vi "ReCalc_V0.11.vi"() -> ()   [LabVIEW 2014]
uses:
  <vilib>/Utility/miscctls.llb/LVPointTypeDef.ctl
  <vilib>/Utility/NIReport.llb/Append Report Text (str wrap).vi
  <vilib>/Utility/xml.llb/Write to XML File(string).vi
  <vilib>/Utility/xml.llb/Read From XML File(string).vi
  <vilib>/Analysis/3filter.llb/IIR Filter (DBL).vi
  <vilib>/Utility/NIReport.llb/NI_report.lvclass
  <vilib>/Analysis/NI_AALPro.lvlib
  <vilib>/Analysis/NI_AALBase.lvlib
panel:
  out "Übersetzung ermitteln aus":T1(ring)
  in  "Datenspeicher":T2
  in  "Speichern":bool
  out "Reifenumfang [m]":dbl=1.222
  out "Getriebe [1:]":dbl=5.343
  out "Zündung [Imp/U]":u8=1
  out "Rolle [Inkr/U]":u16=200
  out "Luftdruck [mbar]":dbl=1013.0
  out "Luftfeuchtigkeit [%]":dbl=50.0
  out "Lufttemperatur [°C]":dbl=20.0
  in  "Berechnen":bool
  in  "Stopp":bool
  in  "Rollenträgheit [kgm²]":dbl=0.402
  in  "Polynom":u8=15
  in  "Gl. Mittelwert":u8=35
  in  "Differenzenquotient":u8=12
  in  "n vom Gas [1/min]":dbl=5000.0
  out "Rollenumfang [m]":dbl=0.613 format="%.3f"
  out "Datum, Zeit":string
  out "Untersetzung aus:":dbl=2.68 format="%.2f"
  in  "Drucken":bool
  out "Pmax":string
  out "Ergebnis":string
  out "Fahrzeugdaten":string
  out "XY-Graph":cluster{dbl[], dbl[]}[](graph)
  in  "Öffnen":bool
  out "korr":dbl
  out "[s]":dbl=5.0
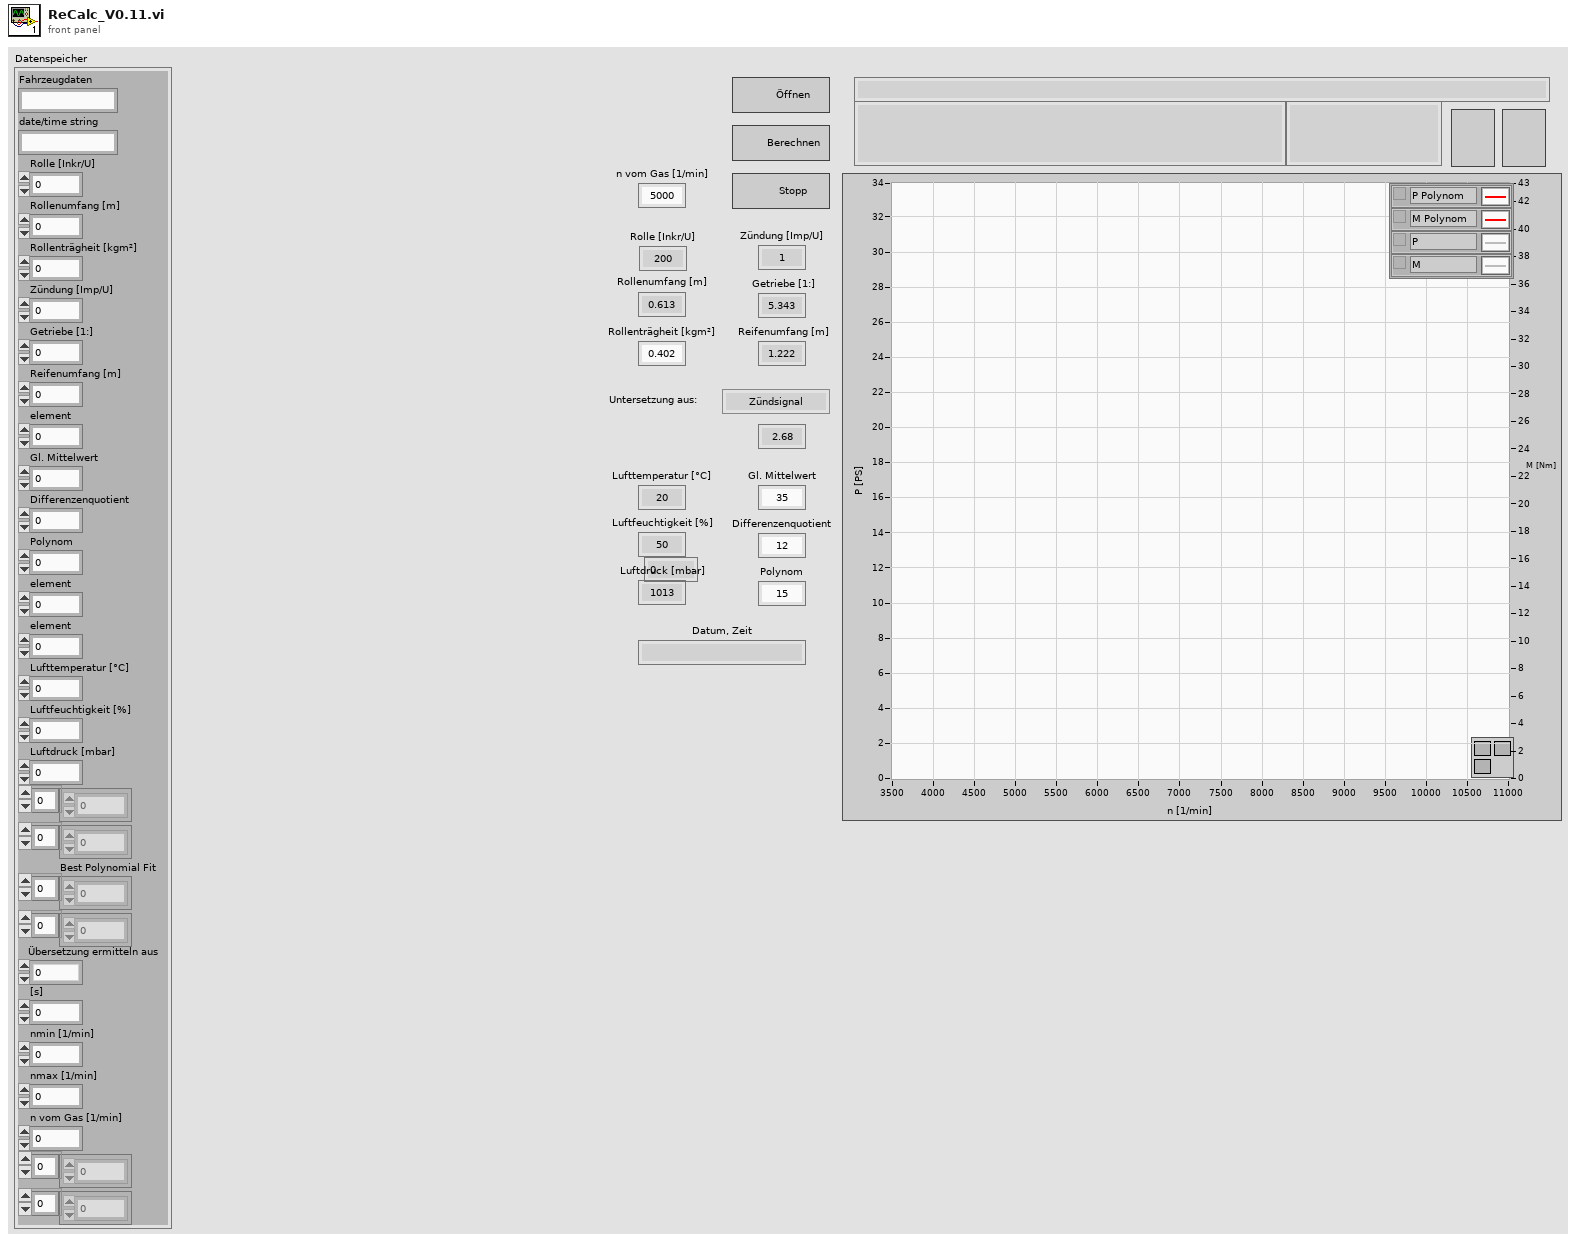
[diagram p1: front panel]
types:
  T1 = enum8{"Zündsignal", "Getriebe & Reifen", "nKuWe / nRolle :"}
  T2 = cluster{"Fahrzeugdaten":string, "date/time string":string, "Rolle [Inkr/U]":u16, "Rollenumfang [m]":dbl, "Rollenträgheit [kgm²]":dbl, "Zündung [Imp/U]":u8, "Getriebe [1:]":dbl, "Reifenumfang [m] ":dbl, "element":dbl, "Gl. Mittelwert":u8, "Differenzenquotient":u8, "Polynom":u8, "element":dbl, "element":dbl, "Lufttemperatur [°C]":dbl, "Luftfeuchtigkeit [%]":dbl, "Luftdruck [mbar]":dbl, dbl[], dbl[], "Best Polynomial Fit":dbl[], dbl[], "Übersetzung ermitteln aus":u8, "[s]":dbl, "nmin [1/min]":dbl, "nmax [1/min]":dbl, "n vom Gas [1/min]":dbl, dbl[], i32[]}
  T3 = typedef "LVPointTypeDef.ctl" = cluster{"Horizontal":i16, "Vertical":i16}
  T4 = enum16{"Kleinste Quadrate", "Kleinestes absolutes Reiduum", "Biquadrat"}
  T5 = cluster{"Fahrzeugdaten":string, "Value":string, "Value":u16, "Value":dbl, "Value":dbl, "Value":u8, "Value":dbl, "Value":dbl, "Value":dbl, "Value":u8, "Value":u8, "Value":u8, "element":dbl, "element":dbl, "Value":dbl, "Value":dbl, "Value":dbl, dbl[], dbl[], "Best Polynomial Fit":dbl[], dbl[], u8, "Value":dbl, dbl, dbl, "Value":dbl, dbl[], i32[]}
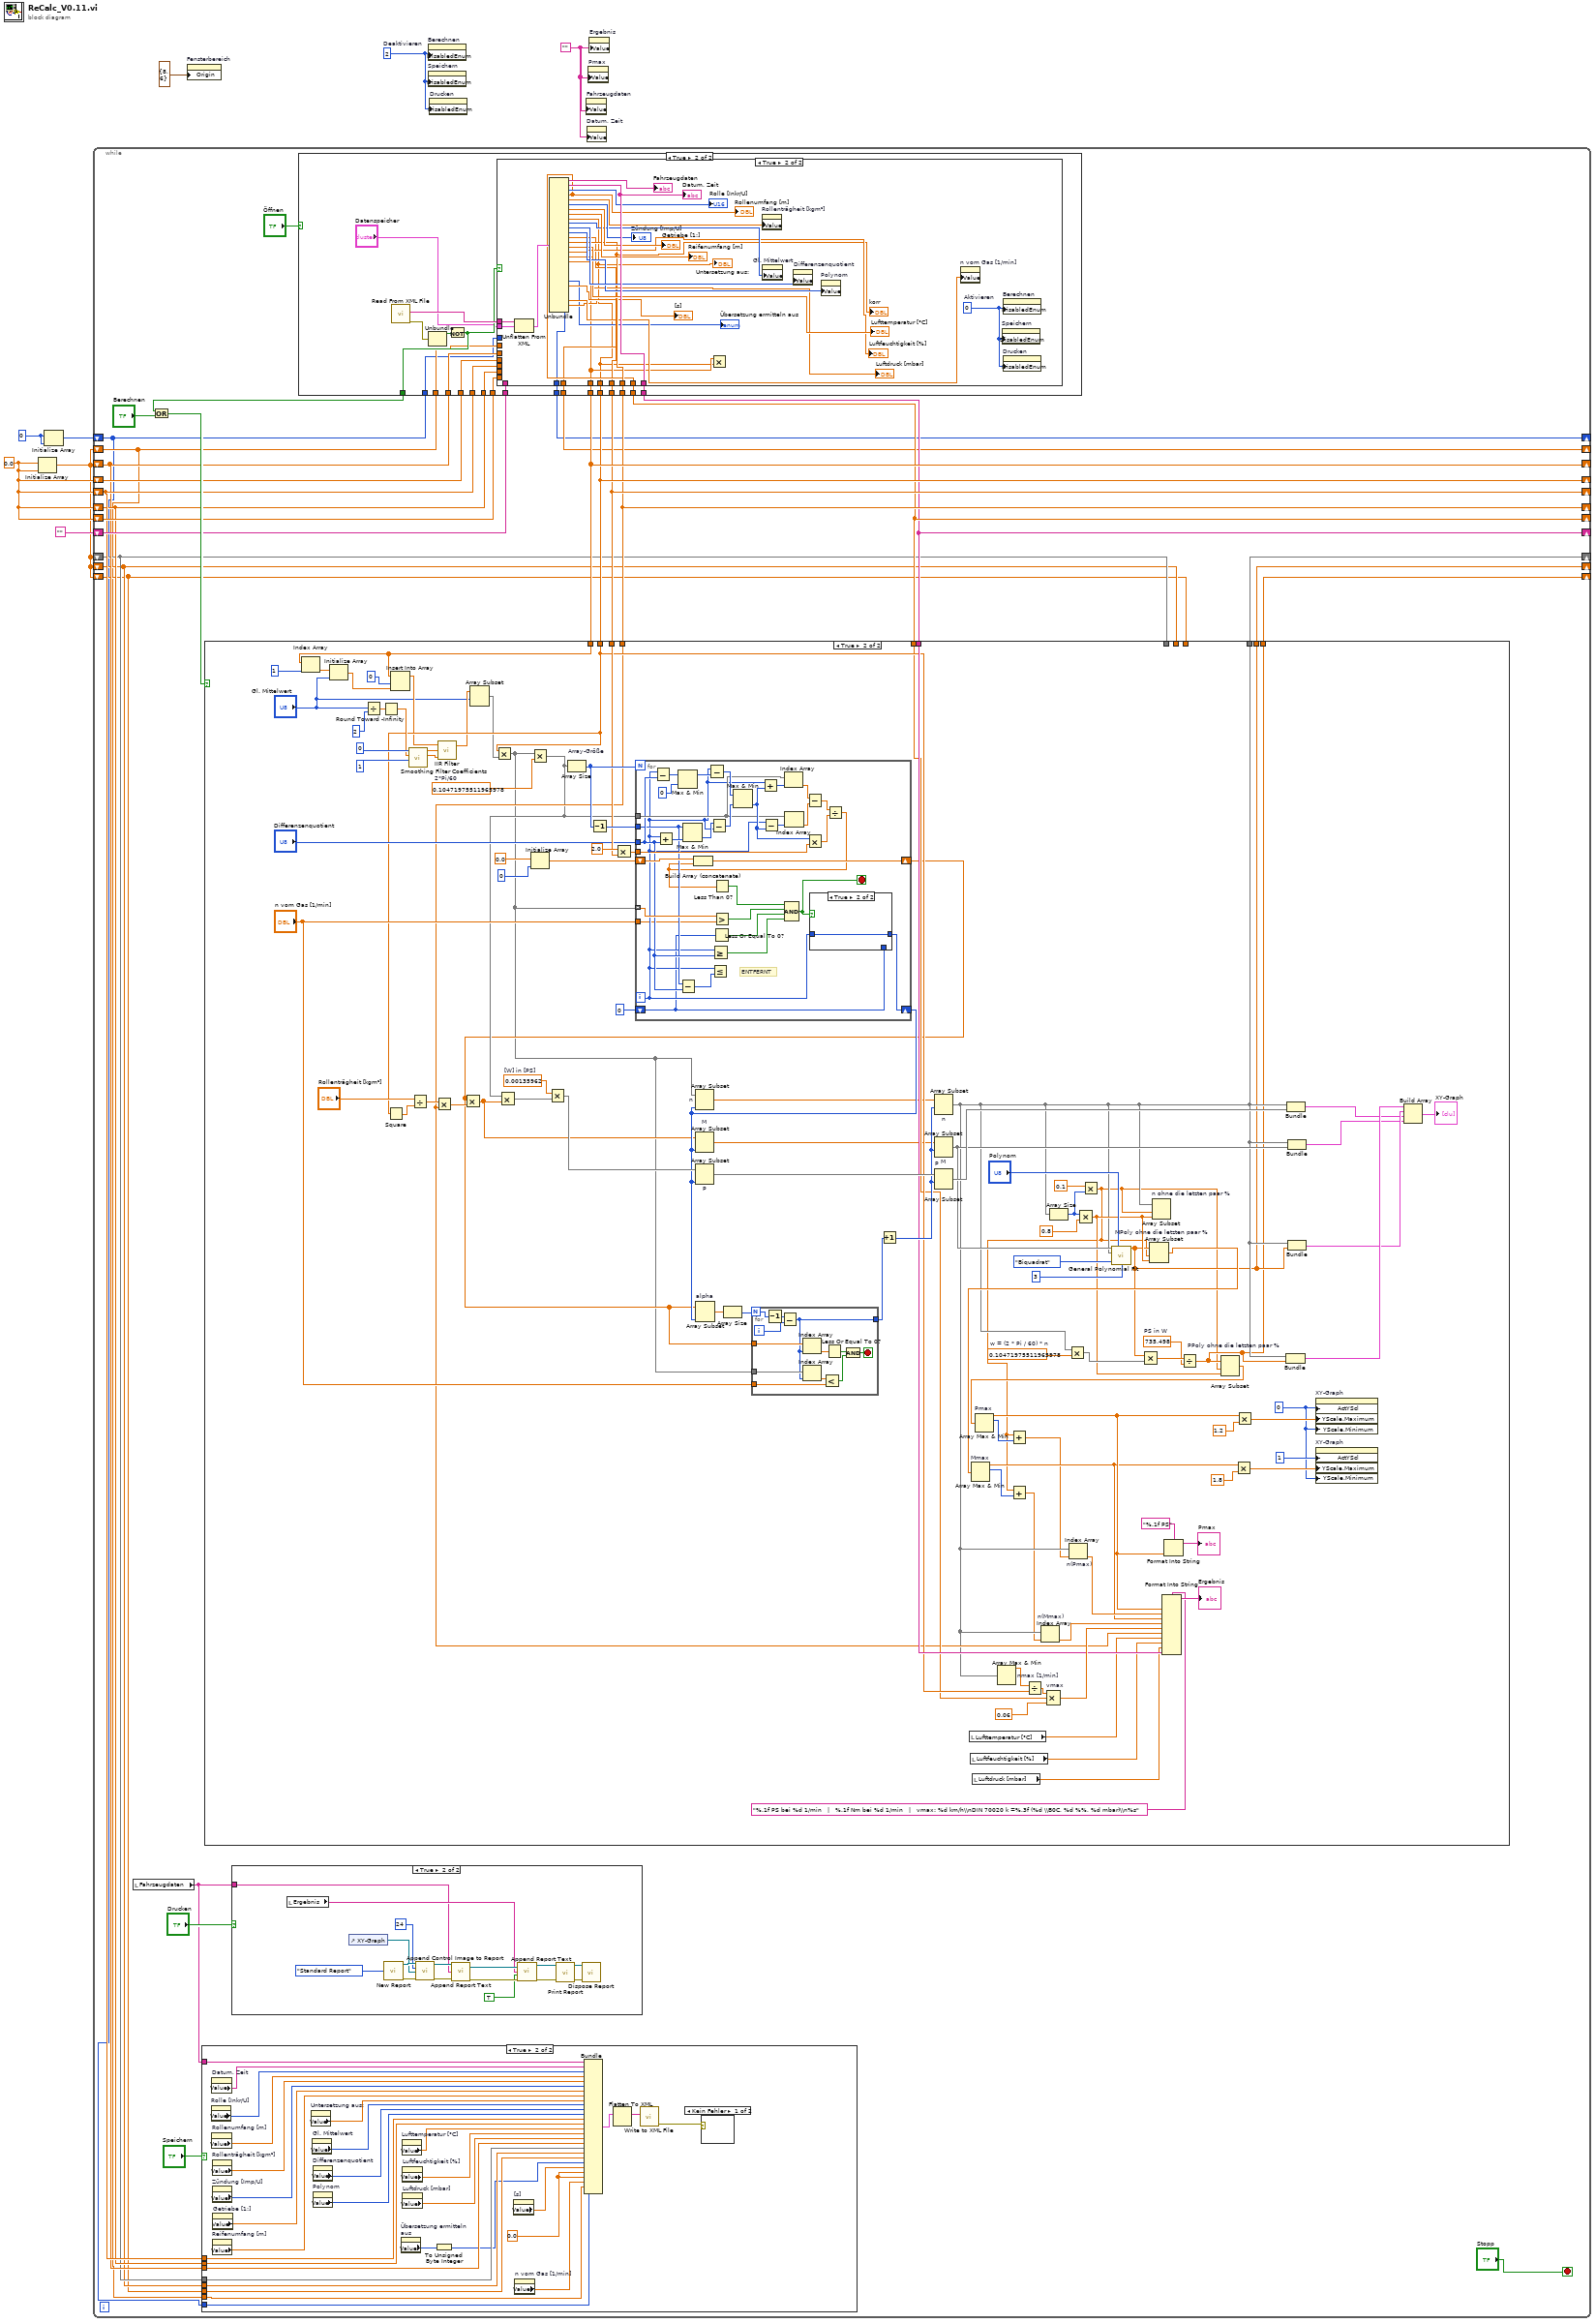
[diagram p0: block diagram]
diagram:
  w1 = 0
  w7 = 0.0
  w4 = 2  # Deaktivieren
  w8 = ""
  n1 = Initialize Array(w7, w7) -> (w3:dbl[])
  n2 = Initialize Array(w1, w1) -> (w2:i32[])
  n3 = while {
    shift-right: [w30] -> _
    shift-left: w3 -> [w19]
    shift-right: [w29] -> _
    shift-left: w7 -> [w33]
    shift-right: [w28] -> _
    shift-left: w7 -> [w21]
    shift-right: [w27] -> _
    shift-left: w7 -> [w20]
    shift-right: [w26] -> _
    shift-left: w7 -> [w32]
    shift-right: [w25] -> _
    shift-left: "" -> [w31]
    shift-right: [w18] -> _
    shift-left: w3 -> [w15]
    shift-right: [w17] -> _
    shift-left: w3 -> [w14]
    shift-right: [w16] -> _
    shift-left: w3 -> [w13]
    shift-right: [w12] -> _
    shift-left: w3 -> [w11]
    shift-right: [w10] -> _
    shift-left: w2 -> [w9]
    stop <- "Stopp" stop-if-true
    n4 = local read "Fahrzeugdaten"() -> (w22:string)
    n5 = case shown="True" "Speichern" {
      tunnel: w22 -> [_ w67]
      tunnel: w21 -> [_ w55]
      tunnel: w20 -> [_ w54]
      tunnel: w19 -> [_ w50]
      tunnel: w15 -> [_ w49]
      tunnel: w14 -> [_ w48]
      tunnel: w13 -> [_ w47]
      tunnel: w11 -> [_ w43]
      tunnel: w9 -> [_ w42]
      frame False {
      }
      frame True {
        w41 = 0.0
        n6 = property on="Rolle [Inkr/U]" class="DigWert (strikt)"() -> ("Value"=w65:u16)  [unwired: 2 in, 2 out]
        n7 = property on="Datum, Zeit" class="Str"() -> ("Value"=w66:string)  [unwired: 2 in, 2 out]
        n8 = property on="Rollenumfang [m]" class="DigWert (strikt)"() -> ("Value"=w64:dbl)  [unwired: 2 in, 2 out]
        n9 = property on="Rollenträgheit [kgm²]" class="DigWert (strikt)"() -> ("Value"=w63:dbl)  [unwired: 2 in, 2 out]
        n10 = property on="Zündung [Imp/U]" class="DigWert (strikt)"() -> ("Value"=w62:u8)  [unwired: 2 in, 2 out]
        n11 = property on="Reifenumfang [m]" class="DigWert (strikt)"() -> ("Value"=w60:dbl)  [unwired: 2 in, 2 out]
        n12 = property on="Getriebe [1:]" class="DigWert (strikt)"() -> ("Value"=w61:dbl)  [unwired: 2 in, 2 out]
        n13 = property on="Untersetzung aus:" class="DigWert (strikt)"() -> ("Value"=w59:dbl)  [unwired: 2 in, 2 out]
        n14 = property on="Gl. Mittelwert" class="DigWert (strikt)"() -> ("Value"=w58:u8)  [unwired: 2 in, 2 out]
        n15 = property on="Differenzenquotient" class="DigWert (strikt)"() -> ("Value"=w57:u8)  [unwired: 2 in, 2 out]
        n16 = property on="Polynom" class="DigWert (strikt)"() -> ("Value"=w56:u8)  [unwired: 2 in, 2 out]
        n17 = property on="Übersetzung ermitteln aus" class="Enum (strikt)"() -> ("Value"=w40:T1)  [unwired: 2 in, 2 out]
        n18 = property on="Lufttemperatur [°C]" class="DigWert (strikt)"() -> ("Value"=w53:dbl)  [unwired: 2 in, 2 out]
        n19 = property on="Luftfeuchtigkeit [%]" class="DigWert (strikt)"() -> ("Value"=w52:dbl)  [unwired: 2 in, 2 out]
        n20 = property on="Luftdruck [mbar]" class="DigWert (strikt)"() -> ("Value"=w51:dbl)  [unwired: 2 in, 2 out]
        n21 = To Unsigned Byte Integer(number=w40) -> (unsigned 8bit integer=w39:u8)
        n22 = property on="[s]" class="DigWert (strikt)"() -> ("Value"=w46:dbl)  [unwired: 2 in, 2 out]
        n23 = property on="n vom Gas [1/min]" class="DigWert (strikt)"() -> ("Value"=w45:dbl)  [unwired: 2 in, 2 out]
        n24 = Bundle("Fahrzeugdaten"=w67, "Value"=w66, "Value"=w65, "Value"=w64, "Value"=w63, "Value"=w62, "Value"=w61, "Value"=w60, "Value"=w59, "Value"=w58, "Value"=w57, "Value"=w56, "element"=w55, "element"=w54, "Value"=w53, "Value"=w52, "Value"=w51, w50, w49, "Best Polynomial Fit"=w48, w47, w39, "Value"=w46, w41, w41, "Value"=w45, w43, w42) -> (w68:T5)  [unwired: 1 in]
        n25 = Flatten To XML(anything=w68) -> (xml string=w69:string)
        n26 = call-poly <vilib>:"Write to XML File.vi"("XML Input"=w69) -> ("error out"=w44:errorcluster)  [unwired: 8 in, 2 out]
        n27 = case shown="Kein Fehler" w44 {
          frame No Error {
          }
          frame Error {
          }
        }
      }
    }
    n28 = case shown="True" "Drucken" {
      tunnel: w22 -> [_ w72]
      frame False {
      }
      frame True {
        n29 = local read "Ergebnis"() -> (w73:string)
        n30 = control-ref of="XY-Graph"() -> (w76:refnum<vi>)
        n31 = call <vilib>:"New Report.vi"("report type"=enum16{"Standard Report", "HTML"}."Standard Report") -> ("report out"=w85:refnum<class "NI_report.lvclass">, "error out"=w84:errorcluster)  [unwired: 13 in]
        n32 = call-dynamic "Append Control Image to Report.vi"("report in"=w85, "image depth"=24, "ctrl reference"=w76, "error in (no error)"=w84) -> ("report out"=w80:refnum<class "NI_report.lvclass">, "error out"=w81:errorcluster)  [unwired: 8 in, 2 out]
        n33 = call-poly <vilib>:"Append Report Text.vi"("report in"=w80, "text"=w72, "error in (no error)"=w81) -> ("report out"=w79:refnum<class "NI_report.lvclass">, "error out"=w78:errorcluster)  [unwired: 9 in, 2 out]
        n34 = call-poly <vilib>:"Append Report Text.vi"("report in"=w79, "text"=w73, "append on new line? (F)"=TRUE, "error in (no error)"=w78) -> ("report out"=w71:refnum<class "NI_report.lvclass">, "error out"=w70:errorcluster)  [unwired: 8 in, 2 out]
        n35 = call-dynamic "Print Report.vi"("report in"=w71, "error in (no error)"=w70) -> ("report out"=w82:refnum<class "NI_report.lvclass">, "error out"=w83:errorcluster)  [unwired: 12 in]
        n36 = call-dynamic "Dispose Report.vi"("report in"=w82, "error in (no error)"=w83) -> ()  [unwired: 13 in, 1 out]
      }
    }
    n37 = case shown="True" "Öffnen" {
      selector: "Öffnen" -> [w243 _]
      tunnel: [w242 w260] -> w30
      tunnel: [w241 w259] -> w29
      tunnel: [w240 w256] -> w28
      tunnel: [w239 w258] -> w27
      tunnel: [w243 w255] -> w37
      tunnel: [w237 w261] -> w25
      tunnel: [w238 w257] -> w26
      tunnel: w19 -> [w242 w254]
      tunnel: w33 -> [w241 w253]
      tunnel: w21 -> [w240 w252]
      tunnel: w20 -> [w239 w250]
      tunnel: w32 -> [w238 w251]
      tunnel: w31 -> [w237 w249]
      tunnel: w11 -> [w236 w248]
      tunnel: [w236 w247] -> w12
      tunnel: [w235 w246] -> w10
      tunnel: w9 -> [w235 w245]
      frame False {
      }
      frame True {
        n38 = call-poly <vilib>:"Read From XML File.vi"() -> ("error out"=w263:errorcluster, "XML Elements"=w264:string)  [unwired: 9 in, 1 out]
        n39 = Unbundle(w263) -> ("status"=w262:bool)  [unwired: 2 out]
        n40 = Not(x=w262) -> (.not. x?=w255:bool)
        n41 = case shown="True" w255 {
          tunnel: w264 -> [_ w299]
          tunnel: "Datenspeicher" -> [_ w298]
          tunnel: [w267 w295] -> w261
          tunnel: [w272 w274] -> w260
          tunnel: [w271 w273] -> w259
          tunnel: [w268 w283] -> w258
          tunnel: [w269 w282] -> w257
          tunnel: [w270 w281] -> w256
          tunnel: w254 -> [w272 _]
          tunnel: w253 -> [w271 _]
          tunnel: w252 -> [w270 _]
          tunnel: w251 -> [w269 _]
          tunnel: w250 -> [w268 _]
          tunnel: w249 -> [w267 _]
          tunnel: w248 -> [w266 _]
          tunnel: [w266 w277] -> w247
          tunnel: [w265 w276] -> w246
          tunnel: w245 -> [w265 _]
          frame False {
          }
          frame True {
            w278 = 0  # Aktivieren
            n42 = Unflatten From XML(xml string=w299, type=w298) -> (value=w297:T2)  [unwired: 1 in, 1 out]
            n43 = Unbundle(w297) -> ("Fahrzeugdaten"=→"Fahrzeugdaten":string, "date/time string"=w295:string, "Rolle [Inkr/U]"=→"Rolle [Inkr/U]":u16, "Rollenumfang [m]"=w282:dbl, "Rollenträgheit [kgm²]"=w292:dbl, "Zündung [Imp/U]"=→"Zündung [Imp/U]":u8, "Getriebe [1:]"=→"Getriebe [1:]":dbl, "Reifenumfang [m]"=→"Reifenumfang [m]":dbl, "element"=w273:dbl, "Gl. Mittelwert"=w289:u8, "Differenzenquotient"=w288:u8, "Polynom"=w287:u8, "element"=w281:dbl, "element"=w283:dbl, "Lufttemperatur [°C]"=→"Lufttemperatur [°C]":dbl, "Luftfeuchtigkeit [%]"=→"Luftfeuchtigkeit [%]":dbl, "Luftdruck [mbar]"=→"Luftdruck [mbar]":dbl, w274:dbl[], "Übersetzung ermitteln aus"=→"Übersetzung ermitteln aus":u8, "[s]"=→"[s]":dbl, "n vom Gas [1/min]"=w279:dbl, w277:dbl[], w276:i32[])  [unwired: 5 out]
            "Datum, Zeit" <- w295
            "Untersetzung aus:" <- w273
            "Rollenumfang [m]" <- w282
            "korr" <- w283
            n44 = Multiply(x=w274, y=w273) -> ()  [unwired: 1 out]
            n45 = property on="Rollenträgheit [kgm²]" class="DigWert (strikt)"("Value"=w292) -> ()  [unwired: 2 in, 2 out]
            n46 = property on="Gl. Mittelwert" class="DigWert (strikt)"("Value"=w289) -> ()  [unwired: 2 in, 2 out]
            n47 = property on="Differenzenquotient" class="DigWert (strikt)"("Value"=w288) -> ()  [unwired: 2 in, 2 out]
            n48 = property on="Polynom" class="DigWert (strikt)"("Value"=w287) -> ()  [unwired: 2 in, 2 out]
            n49 = property on="n vom Gas [1/min]" class="DigWert (strikt)"("Value"=w279) -> ()  [unwired: 2 in, 2 out]
            n50 = property on="Speichern" class="Bool."("DisabledEnum"=w278) -> ()  [unwired: 2 in, 2 out]
            n51 = property on="Berechnen" class="Bool."("DisabledEnum"=w278) -> ()  [unwired: 2 in, 2 out]
            n52 = property on="Drucken" class="Bool."("DisabledEnum"=w278) -> ()  [unwired: 2 in, 2 out]
          }
        }
      }
    }
    n53 = Or(x=w37, y="Berechnen") -> (x .or. y?=w35:bool)
    n54 = case shown="True" w35 {
      tunnel: w30 -> [_ w91]
      tunnel: w28 -> [_ w169]
      tunnel: w25 -> [_ w136]
      tunnel: w29 -> [_ w135]
      tunnel: w26 -> [_ w134]
      tunnel: w27 -> [_ w133]
      tunnel: [w88 w109] -> w18
      tunnel: [w87 w108] -> w17
      tunnel: [w86 w107] -> w16
      tunnel: w15 -> [w88 _]
      tunnel: w14 -> [w87 _]
      tunnel: w13 -> [w86 _]
      frame False {
      }
      frame True {
        w145 = 0
        w154 = 735.498  # PS in W
        w159 = 0.10471975511965978  # w = (2 * Pi / 60) * n
        w174 = 0.00135962  # [W] in [PS]
        w183 = 0.10471975511965978  # 2*Pi/60
        n55 = Index Array(array=w91, index=1) -> (element=w96:dbl)
        n56 = Initialize Array(w96, "Gl. Mittelwert") -> (w97:dbl[])
        n57 = Divide(x="Gl. Mittelwert", y=2) -> (x/y=w186:dbl)
        n58 = Round Toward -Infinity(1:w186) -> (0:w185:dbl)
        n59 = Square(x=w135) -> (x^2=w175:dbl)
        n60 = Insert Into Array ("In Array einfügen")(array=w91, index=0, new element=w97) -> (w94:dbl[])
        n61 = call <vilib>:"Smoothing Filter Coefficients.vi"("shape"=1, "half-width"=w185, "type"=0) -> ("forward coefficients"=w98:dbl[], "reverse coefficients"=w99:dbl[])  [unwired: 6 in, 1 out]
        n62 = Divide(x="Rollenträgheit [kgm²]", y=w175) -> (x/y=w172:dbl)
        n63 = Multiply(x=w172, y=w133) -> (x*y=w171:dbl)
        n64 = call-poly <vilib>:"IIR Filter.vi"("Forward Coefficients"=w98, "Reverse Coefficients"=w99, "X"=w94) -> ("Filtered X"=w93:dbl[])  [unwired: 1 in, 1 out]
        n65 = Array Subset(array=w93, index="Gl. Mittelwert") -> (w90:dbl[])  [unwired: 1 in]
        n66 = Multiply(x=w135, y=w90) -> (x*y=w101:dbl[])
        n67 = Multiply(x=w101, y=w183) -> (x*y=w128:dbl[])
        n68 = Initialize Array(0.0 ("y"), 0) -> (w176:dbl[])
        n69 = Array Size "Array-Größe"(array=w128) -> (size(s)=w181:i32)
        n70 = Decrement(x=w181) -> (x-1=w182:i32)
        n71 = Multiply(x=2.0, y=w169) -> (x*y=w180:dbl)
        n72 = for {
          N: w181 -> [_]
          tunnel: "Differenzenquotient" -> [w211]
          tunnel: w128 -> [w218]
          tunnel: w182 -> [w210]
          tunnel: w180 -> [w219]
          shift-right: [w215] -> w127
          shift-left: w176 -> [w216]
          tunnel: w101 -> [w213] mode=indexing
          tunnel: "n vom Gas [1/min]" -> [w202]
          shift-right: [w201] -> w164
          shift-left: 0 -> [w204]
          i -> [w205]
          stop <- w203 stop-if-true
          # "ENTFERNT"
          n73 = Subtract(x=w205, y=w211) -> (x-y=w232:i32)
          n74 = Add(x=w205, y=w211) -> (x+y=w226:i32)
          n75 = Max & Min(x=w232, y=0) -> (max(x,y)=w230:i32)  [unwired: 1 out]
          n76 = Subtract(x=w210, y=w211) -> (x-y=w212:i32)
          n77 = Max & Min(x=w210, y=w226) -> (min(x,y)=w227:i32)  [unwired: 1 out]
          n78 = Subtract(x=w205, y=w230) -> (x-y=w229:i32)
          n79 = Subtract(x=w227, y=w205) -> (x-y=w228:i32)
          n80 = Less Or Equal?(x=w205, y=w212) -> ()  [unwired: 1 out]
          n81 = Greater Or Equal?(x=w205, y=w211) -> (x >= y?=w208:bool)
          n82 = Less Or Equal To 0?(x=w204) -> (x <= 0?=w206:bool)
          n83 = Greater?(x=w213, y=w202) -> (0:w214:bool)
          n84 = Max & Min(x=w229, y=w228) -> (min(x,y)=w220:i32)  [unwired: 1 out]
          n85 = Add(x=w205, y=w220) -> (x+y=w225:i32)
          n86 = Subtract(x=w205, y=w220) -> (x-y=w224:i32)
          n87 = Index Array(array=w218, index=w225) -> (element=w222:dbl)
          n88 = Index Array(array=w218, index=w224) -> (element=w223:dbl)
          n89 = Subtract(x=w222, y=w223) -> (x-y=w221:dbl)
          n90 = Multiply(x=w220, y=w219) -> (x*y=w217:dbl)
          n91 = Divide(x=w221, y=w217) -> (x/y=w209:dbl)
          n92 = Build Array (concatenate)(w216, w209) -> (w215:dbl[])
          n93 = Less Than 0?(x=w209) -> (x < 0?=w207:bool)
          n94 = Compound Arithmetic op=AND(w207, w214, w206, w208) -> (w203:bool)
          n95 = case shown="True" w203 {
            tunnel: w205 -> [_ w234]
            tunnel: [w233 w234] -> w201
            tunnel: w204 -> [w233 _]
            frame False {
            }
            frame True {
            }
          }
        }
        n96 = Multiply(x=w127, y=w171) -> (x*y=w125:dbl[])
        n97 = Multiply(x=w128, y=w125) -> (x*y=w173:dbl[])
        n98 = Multiply(x=w174, y=w173) -> (x*y=w165:dbl[])
        n99 = Array Subset "n"(array=w101, length=w164) -> (w100:dbl[])  [unwired: 1 in]
        n100 = Array Subset "M"(array=w125, length=w164) -> (w126:dbl[])  [unwired: 1 in]
        n101 = Array Subset "P"(array=w165, length=w164) -> (w153:dbl[])  [unwired: 1 in]
        n102 = Array Subset "alpha"(array=w127, length=w164) -> (w166:dbl[])  [unwired: 1 in]
        n103 = Array Size(array=w166) -> (size(s)=w163:i32)
        n104 = for {
          N: w163 -> [w200]
          tunnel: w127 -> [w197]
          tunnel: w101 -> [w194]
          tunnel: "n vom Gas [1/min]" -> [w191]
          tunnel: [w189] -> w161
          i -> [w195]
          stop <- w190 stop-if-true
          n105 = Decrement(x=w200) -> (x-1=w199:i32)
          n106 = Subtract(x=w199, y=w195) -> (x-y=w189:i32)
          n107 = Index Array(array=w197, index=w189) -> (element=w198:dbl)
          n108 = Index Array(array=w194, index=w189) -> (element=w193:dbl)
          n109 = Less?(x=w193, y=w191) -> (x < y?=w192:bool)
          n110 = Less Or Equal To 0?(x=w198) -> (x <= 0?=w196:bool)
          n111 = And(x=w196, y=w192) -> (x .and. y?=w190:bool)
        }
        n112 = Increment(x=w161) -> (x+1=w152:i32)
        n113 = Array Subset "n"(array=w100, index=w152) -> (w109:dbl[])  [unwired: 1 in]
        n114 = Array Subset "M"(array=w126, index=w152) -> (w158:dbl[])  [unwired: 1 in]
        n115 = Array Subset "P"(array=w153, index=w152) -> (w160:dbl[])  [unwired: 1 in]
        n116 = local read "Lufttemperatur [°C]"() -> (w118:dbl)
        n117 = local read "Luftfeuchtigkeit [%]"() -> (w116:dbl)
        n118 = local read "Luftdruck [mbar]"() -> (w117:dbl)
        n119 = Array Max & Min "nmax [1/min]"(array=w109) -> (max value=w143:dbl)  [unwired: 3 out]
        n120 = Divide(x=w143, y=w135) -> (x/y=w142:dbl)
        n121 = Compound Arithmetic op=MULTIPLY "vmax"(w142, w134, 0.06) -> (w138:dbl)
        n122 = Array Size(array=w109) -> (size(s)=w111:i32)
        n123 = Multiply(x=w109, y=w159) -> (x*y=w144:dbl[])
        n124 = Multiply(x=w111, y=0.8) -> (x*y=w112:dbl)
        n125 = Multiply(x=0.1, y=w111) -> (x*y=w104:dbl)
        n126 = call <vilib>:"General Polynomial Fit.vi"("Y"=w158, "polynomial order"="Polynom", "X"=w109, "method"=T4."Biquadrat" ("Methode"), "algorithm"=3) -> ("Best Polynomial Fit"=w108:dbl[])  [unwired: 7 in, 3 out]
        n127 = Multiply(x=w108, y=w144) -> (x*y=w155:dbl[])
        n128 = Array Subset "MPoly ohne die letzten paar %"(array=w108, index=w104, length=w112) -> (w113:dbl[])
        n129 = Array Max & Min "Mmax"(array=w113) -> (max value=w131:dbl, max index (indices)=w105:i32)  [unwired: 2 out]
        n130 = Add(x=w104, y=w105) -> (x+y=w103:dbl)
        n131 = Index Array "n(Mmax)"(array=w109, index=w103) -> (element=w139:dbl)
        n132 = Array Subset "n ohne die letzten paar %"(array=w109, index=w104, length=w112) -> ()  [unwired: 1 out]
        n133 = Divide(x=w155, y=w154) -> (x/y=w107:dbl[])
        n134 = Array Subset "PPoly ohne die letzten paar %"(array=w107, index=w104, length=w112) -> (w114:dbl[])
        n135 = Array Max & Min "Pmax"(array=w114) -> (max value=w132:dbl, max index (indices)=w106:i32)  [unwired: 2 out]
        n136 = Add(x=w104, y=w106) -> (x+y=w102:dbl)
        n137 = Index Array "n(Pmax)"(array=w109, index=w102) -> (element=w140:dbl)
        n138 = Format Into String(format string="%.1f PS bei %d 1/min   |   %.1f Nm bei %d 1/min   |   vmax: %d km/h\\nDIN 70020 k =%.3f (%d \\B0C, %d %%, %d mbar)\\n%s" ("Format-String"), w132, w140, w131, w139, w138, w133, w118, w116, w117, w136) -> (resulting string=→"Ergebnis":string)  [unwired: 2 in, 1 out]
        n139 = Format Into String(format string="%.1f PS" ("Format-String"), w132) -> (resulting string=→"Pmax":string)  [unwired: 2 in, 1 out]
        n140 = Multiply(x=w131, y=1.8) -> (x*y=w146:dbl)
        n141 = Multiply(x=w132, y=1.2) -> (x*y=w147:dbl)
        n142 = Bundle(w109, w107) -> (w123:cluster{dbl[], dbl[]})  [unwired: 1 in]
        n143 = Bundle(w109, w160) -> (w121:cluster{dbl[], dbl[]})  [unwired: 1 in]
        n144 = Bundle(w109, w158) -> (w120:cluster{dbl[], dbl[]})  [unwired: 1 in]
        n145 = Bundle(w109, "Best Polynomial Fit"=w108) -> (w122:cluster{dbl[], "Best Polynomial Fit":dbl[]})  [unwired: 1 in]
        n146 = property on="XY-Graph" class="XYGraph (strikt)"("ActYScl"=w145, "YScale.Maximum"=w147, "YScale.Minimum"=w145) -> ()  [unwired: 2 in, 2 out]
        n147 = property on="XY-Graph" class="XYGraph (strikt)"("ActYScl"=1, "YScale.Maximum"=w146, "YScale.Minimum"=w145) -> ()  [unwired: 2 in, 2 out]
        n148 = Build Array(w123, w122, w121, w120) -> (→"XY-Graph":cluster{dbl[], "Best Polynomial Fit":dbl[]}[])
      }
    }
  }
  n149 = property on="Fensterbereich" class="Bereich"("Origin"=T3 {"Horizontal"=8, "Vertical"=6}) -> ()  [unwired: 2 in, 2 out]
  n150 = property on="Berechnen" class="Bool."("DisabledEnum"=w4) -> ()  [unwired: 2 in, 2 out]
  n151 = property on="Speichern" class="Bool."("DisabledEnum"=w4) -> ()  [unwired: 2 in, 2 out]
  n152 = property on="Drucken" class="Bool."("DisabledEnum"=w4) -> ()  [unwired: 2 in, 2 out]
  n153 = property on="Fahrzeugdaten" class="Str"("Value"=w8) -> ()  [unwired: 2 in, 2 out]
  n154 = property on="Datum, Zeit" class="Str"("Value"=w8) -> ()  [unwired: 2 in, 2 out]
  n155 = property on="Pmax" class="Str"("Value"=w8) -> ()  [unwired: 2 in, 2 out]
  n156 = property on="Ergebnis" class="Str"("Value"=w8) -> ()  [unwired: 2 in, 2 out]
